vi "yokogawa_com.vi"() -> ()   [LabVIEW 2011]
panel:
  out "Waveform Graph":cluster{"start":dbl, "delt":dbl, "Output":dbl[]}(graph)
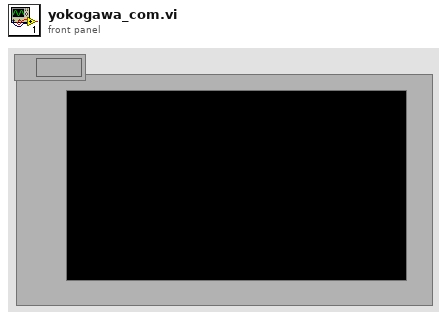
[diagram p1: front panel]
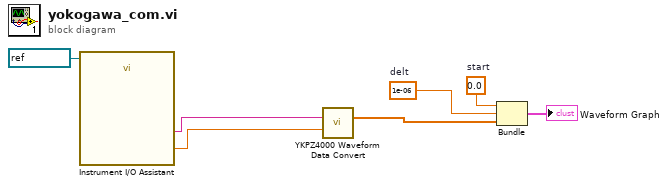
[diagram p0: block diagram]
diagram:
  w3 = 1e-06  # delt
  w5 = 0.0  # start
  n1 = call "Instrument I/O Assistant"("Session In"=refnum<visa-resource-name> "COM1") -> ("ouput"=w6:string, "range"=w7:dbl)  [unwired: 23 in, 2 out]
  n2 = call <instrlib>:"YKPZ4000 Waveform Data Convert.vi"("Input Data"=w6, "Range"=w7) -> ("Output"=w2:dbl[])  [unwired: 11 in, 2 out]
  n3 = Bundle("start"=w5, "delt"=w3, "Output"=w2) -> (→"Waveform Graph":cluster{"start":dbl, "delt":dbl, "Output":dbl[]})  [unwired: 1 in]
